vi "后台服务.vi"() -> ()   [LabVIEW 2016, in "仿真数据.lvlib"]
panel:
  out "范围内？":bool
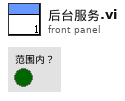
[diagram p1: front panel]
types:
  T1 = enum16{"00", "01", "02", "03", "04", "05", "06", "07", "08", "09", "10", "11", "12", "13", "14", "15", "16", "17", "18", "19", "20", "21", "22", "23", "关闭"}
  T2 = enum16{"00", "01", "02", "03", "04", "05", "06", "07", "08", "09", "10", "11", "12", "13", "14", "15", "16", "17", "18", "19", "20", "21", "22", "23"}
  T3 = typedef "LVDateTimeRec.ctl" = cluster{"秒数的小数部分":dbl, "秒":i32, "分":i32, "时":i32, "日":i32, "月":i32, "年":i32, "天数（周）":i32, "天数（年）":i32, "DST":i32}
  T4 = cluster{"切换阈值":dbl, "稳定系数":dbl, "变异系数":dbl, "enable":bool, "init":bool}
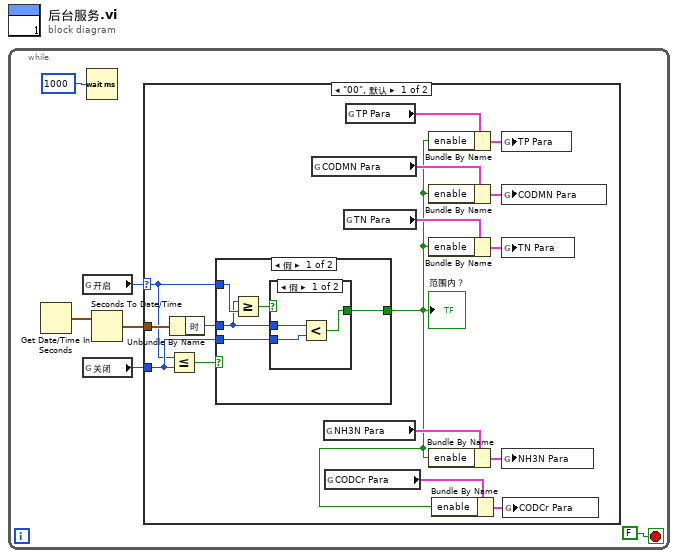
[diagram p0: block diagram]
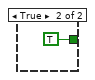
[diagram p2: hidden frame]
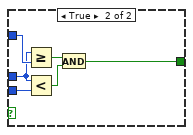
[diagram p3: hidden frame]
diagram:
  n1 = while {
    stop <- FALSE stop-if-true
    n2 = Get Date/Time In Seconds() -> (seconds since 1Jan1904=w3:timestamp)
    n3 = global read "仿真全局变量.vi" "开启"() -> (w6:T1)
    n4 = global read "仿真全局变量.vi" "关闭"() -> (w4:T2)
    n5 = Wait (ms)(milliseconds to wait=u32 1000 ("等待时间（毫秒）")) -> ()  [unwired: 1 out]
    n6 = Seconds To Date/Time(time stamp (now)=w3) -> (date time rec=w5:T3)  [unwired: 1 in]
    n7 = case shown="\"00\", 默认" w6 {
      selector: w6 -> [w18 _]
      tunnel: w5 -> [w22 _]
      tunnel: w4 -> [w19 _]
      frame "00", Default {
        n8 = Less Or Equal?(x=w18, y=w19) -> (x <= y?=w21:bool)
        n9 = Unbundle By Name(w22) -> ("时"=w20:i32)
        n10 = case shown="假" w21 {
          tunnel: w20 -> [w25 w36]
          tunnel: w19 -> [w24 w35]
          tunnel: w18 -> [w27 w37]
          tunnel: [w23 w32] -> w7
          frame False {
            n11 = Greater Or Equal?(x=w25, y=w27) -> (x >= y?=w26:bool)
            n12 = case shown="假" w26 {
              tunnel: [w28 TRUE] -> w23
              tunnel: w25 -> [w30 _]
              tunnel: w24 -> [w29 _]
              frame False {
                n13 = Less?(x=w30, y=w29) -> (x < y?=w28:bool)
              }
              frame True {
              }
            }
          }
          frame True {
            n14 = Greater Or Equal?(x=w36, y=w37) -> (x >= y?=w33:bool)
            n15 = Less?(x=w36, y=w35) -> (x < y?=w34:bool)
            n16 = And(x=w33, y=w34) -> (x .and. y?=w32:bool)
          }
        }
        "范围内？" <- w7
        n17 = global read "仿真全局变量.vi" "CODMN Para"() -> (w17:T4)
        n18 = global read "仿真全局变量.vi" "NH3N Para"() -> (w10:T4)
        n19 = global read "仿真全局变量.vi" "CODCr Para"() -> (w9:T4)
        n20 = global read "仿真全局变量.vi" "TN Para"() -> (w13:T4)
        n21 = global read "仿真全局变量.vi" "TP Para"() -> (w14:T4)
        n22 = Bundle By Name(cluster=w14, "enable"=w7) -> (w15:T4)
        n23 = Bundle By Name(cluster=w17, "enable"=w7) -> (w16:T4)
        n24 = Bundle By Name(cluster=w13, "enable"=w7) -> (w12:T4)
        n25 = Bundle By Name(cluster=w10, "enable"=w7) -> (w11:T4)
        n26 = Bundle By Name(cluster=w9, "enable"=w7) -> (w8:T4)
        n27 = global write "仿真全局变量.vi" "TP Para"(w15) -> ()
        n28 = global write "仿真全局变量.vi" "CODMN Para"(w16) -> ()
        n29 = global write "仿真全局变量.vi" "TN Para"(w12) -> ()
        n30 = global write "仿真全局变量.vi" "NH3N Para"(w11) -> ()
        n31 = global write "仿真全局变量.vi" "CODCr Para"(w8) -> ()
      }
      frame "关闭" {
      }
    }
  }
